vi "_create_metadata_and_aliases.vi"(8 "error in":errorcluster) -> (0 "error out":errorcluster, 4 "log":string)   [LabVIEW 2024]
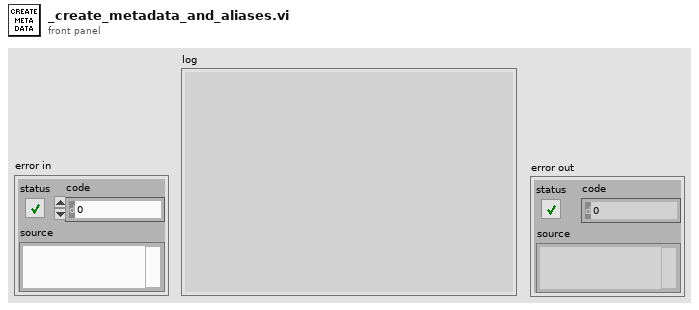
[diagram p1: front panel]
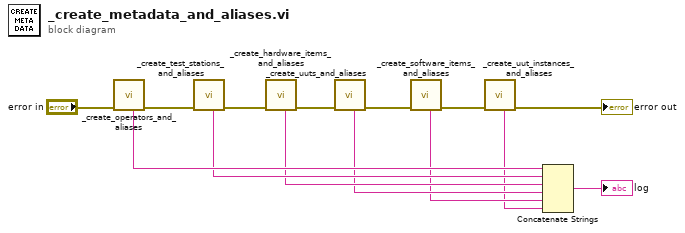
[diagram p0: block diagram]
diagram:
  n1 = call "_create_operators_and_aliases.vi"("error in"="error in") -> ("error out"=w14:errorcluster, "log"=w7:string)  [unwired: 9 in]
  n2 = call "_create_test_stations_and_aliases.vi"("error in"=w14) -> ("error out"=w13:errorcluster, "log"=w6:string)  [unwired: 9 in]
  n3 = call "_create_hardware_items_and_aliases.vi"("error in"=w13) -> ("error out"=w12:errorcluster, "log"=w5:string)  [unwired: 9 in]
  n4 = call "_create_uuts_and_aliases.vi"("error in"=w12) -> ("error out"=w11:errorcluster, "log"=w4:string)  [unwired: 9 in]
  n5 = call "_create_software_items_and_aliases.vi"("error in"=w11) -> ("error out"=w9:errorcluster, "log"=w3:string)  [unwired: 9 in]
  n6 = call "_create_uut_instances_and_aliases.vi"("error in"=w9) -> ("error out"=→"error out":errorcluster, "log"=w2:string)  [unwired: 9 in]
  n7 = Concatenate Strings(w7, w6, w5, w4, w3, w2) -> (→"log":string)
